vi "Parse All Elements.vi"(0 "Node in":refnum<k20>, 11 "error in":errorcluster) -> (4 "Node out":refnum<k20>, 6 "Section Data":T1, 8 "Child Items":cluster{"Item Type":T2, "Value":variant}[](array[cluster]), 10 "Properties out":refnum<class "Property.lvclass">[](array[class]), 15 "error out":errorcluster)   [LabVIEW 2024, in "Parser.lvlib" / "Section.lvclass"]
uses:
  Section.lvclass
  Item/Controls/Item Type.ctl
  Property/Property.lvclass
  <vilib>/xml/Close Reference(Node).vi
  <resource>/objmgr/DOMUserDefRef.rc
  <vilib>/xml/NI_XML.lvlib
  Channel/Channel.lvclass
  Item/Item.lvclass
  Parser.lvlib
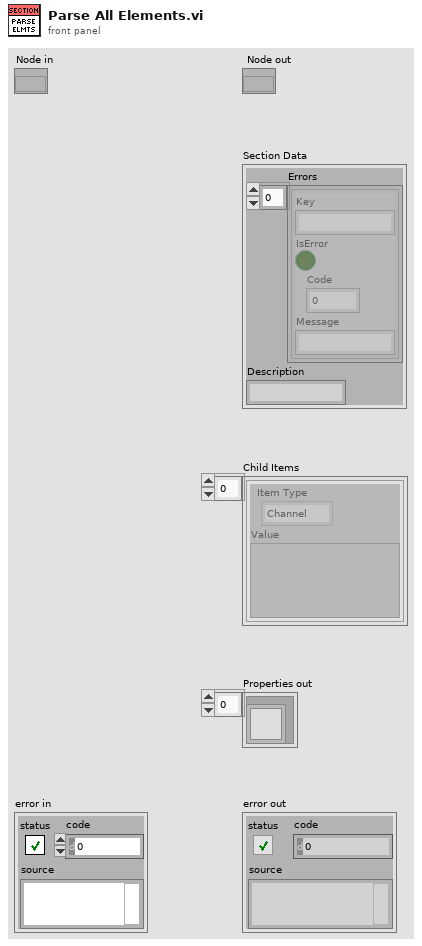
[diagram p1: front panel]
types:
  T1 = cluster{"Errors":cluster{"Key":string, "IsError":bool, "Code":u32, "Message":string}[], "Description":string}
  T2 = typedef "Parser.lvlib/Item.lvclass/Item Type.ctl" = enum16{"Channel", "Section"}
  T3 = cluster{"Key":string, "IsError":bool, "Code":u32, "Message":string}[]
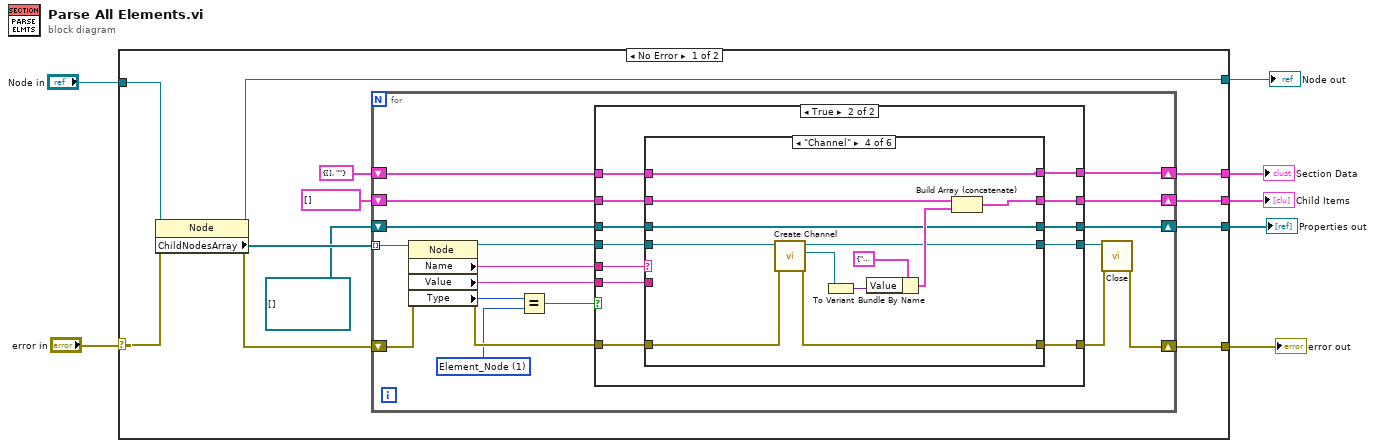
[diagram p0: block diagram]
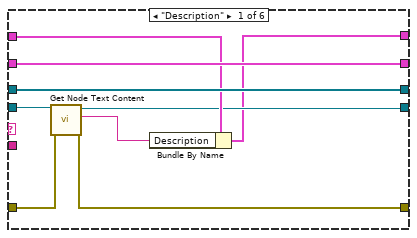
[diagram p3: hidden frame]
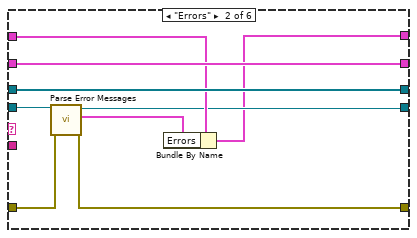
[diagram p4: hidden frame]
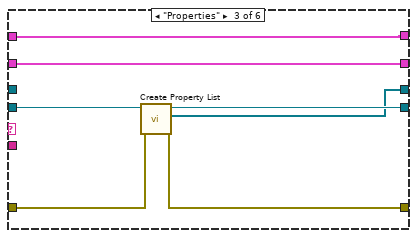
[diagram p5: hidden frame]
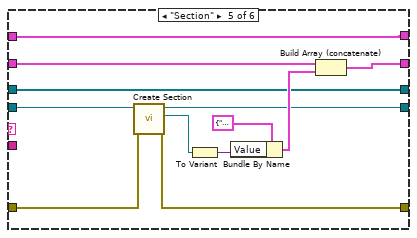
[diagram p6: hidden frame]
diagram:
  n1 = case shown="No Error" "error in" {
    selector: "error in" -> [w17 w109]
    tunnel: [w18 w109] -> w7
    tunnel: "Node in" -> [w16 _]
    tunnel: [w13 _] -> w4
    tunnel: [w11 _] -> w3
    tunnel: [w9 _] -> w2
    tunnel: [w8 _] -> w1
    frame No Error {
      n2 = property class="Node"(reference=w16, error in=w17) -> (reference out=w8:refnum<k20>, error out=w19:errorcluster, "ChildNodesArray"=w15:refnum<k20>[])
      n3 = for {
        tunnel: w15 -> [w33] mode=indexing
        shift-right: [w36] -> w18
        shift-left: w19 -> [w37]
        shift-right: [w24] -> w9
        shift-left: T1 {"Errors"=[], "Description"=""} ("Cluster of class private data") -> [w25]
        shift-right: [w22] -> w13
        shift-left: cluster{"Item Type":T2, "Value":variant}[] [] ("Child Items") -> [w23]
        shift-right: [w20] -> w11
        shift-left: refnum<class "Property.lvclass">[] [] ("reference out") -> [w21]
        w28 = 1 items=["Element_Node"=1, "Attribute_Node"=2, "Text_Node"=3, "CDATASection_Node"=4, "EntityReference_Node"=5, "Entity_Node"=6, "ProcessingInstruction_Node"=7, "Comment_Node"=8, "Document_Node"=9, "DocumentType_Node"=10, "DocumentFragment_Node"=11, "Notation_Node"=12] ("Node Type")
        n4 = property on="Property Node" class="Node"(reference=w33, error in=w37) -> (reference out=w31:refnum<k20>, error out=w35:errorcluster, "Name"=w32:string, "Value"=w30:string, "Type"=w26:i32)
        n5 = Equal?(x=w26, y=w28) -> (x = y?=w27:bool)
        n6 = case shown="True" w27 {
          tunnel: w32 -> [_ w52]
          tunnel: w31 -> [w41 w51]
          tunnel: w30 -> [_ w50]
          tunnel: [w41 w49] -> w29
          tunnel: w35 -> [w42 w54]
          tunnel: [w42 w53] -> w34
          tunnel: w25 -> [w40 w48]
          tunnel: [w40 w47] -> w24
          tunnel: w23 -> [w39 w46]
          tunnel: [w39 w45] -> w22
          tunnel: w21 -> [w38 w44]
          tunnel: [w38 w43] -> w20
          frame False {
          }
          frame True {
            n7 = case shown="\"Channel\"" w52 {
              tunnel: w51 -> [w58 w67 w77 w88 w100 w107]
              tunnel: w50 -> [_ _ _ _ _ _]
              tunnel: [w56 w66 w76 w80 w92 w107] -> w49
              tunnel: w54 -> [w63 w72 w79 w91 w103 w108]
              tunnel: [w62 w71 w78 w90 w102 w108] -> w53
              tunnel: w48 -> [w59 w68 w75 w89 w101 w106]
              tunnel: [w55 w64 w75 w89 w101 w106] -> w47
              tunnel: w46 -> [w61 w70 w73 w85 w97 w104]
              tunnel: [w61 w70 w73 w83 w95 w104] -> w45
              tunnel: w44 -> [w60 w69 _ w82 w94 w105]
              tunnel: [w60 w69 w74 w82 w94 w105] -> w43
              frame "Description" {
                n8 = call <vilib>:"Get Node Text Content.vi"("error in (no error)"=w63, "node in"=w58) -> ("error out"=w62:errorcluster, "node text"=w57:string, "node out"=w56:refnum<k20>)  [unwired: 7 in]
                n9 = Bundle By Name(cluster=w59, "Description"=w57) -> (w55:T1)
              }
              frame "Errors" {
                n10 = call "Parse Error Messages.vi"("error in"=w72, "Node in"=w67) -> ("error out"=w71:errorcluster, "Errors"=w65:T3, "Node out"=w66:refnum<k20>)  [unwired: 7 in]
                n11 = Bundle By Name(cluster=w68, "Errors"=w65) -> (w64:T1)
              }
              frame "Properties" {
                n12 = call "Create Property List.vi"("error in"=w79, "Property Nodes In"=w77) -> ("error out"=w78:errorcluster, "Properties out"=w74:refnum<class "Property.lvclass">[], "Property Nodes out"=w76:refnum<k20>)  [unwired: 7 in]
              }
              frame "Channel" {
                n13 = call "Create Channel.vi"("error in"=w91, "Node In"=w88) -> ("error out"=w90:errorcluster, "Channel out"=w81:refnum<class "Channel.lvclass">, "Node out"=w80:refnum<k20>)  [unwired: 7 in]
                n14 = To Variant(anything=w81) -> (Variant=w86:variant)
                n15 = Bundle By Name(cluster=cluster{"Item Type":T2, "Value":variant} {"Item Type"=enum."Channel", "Value"=variant} ("Child Items"), "Value"=w86) -> (w84:cluster{"Item Type":T2, "Value":variant})
                n16 = Build Array (concatenate)(w85, w84) -> (w83:cluster{"Item Type":T2, "Value":variant}[])
              }
              frame "Section" {
                n17 = call "Create Section.vi"("error in"=w103, "Node In"=w100) -> ("error out"=w102:errorcluster, "Section out"=w93:refnum<class "Section.lvclass">, "Node out"=w92:refnum<k20>)  [unwired: 7 in]
                n18 = To Variant(anything=w93) -> (Variant=w98:variant)
                n19 = Bundle By Name(cluster=cluster{"Item Type":T2, "Value":variant} {"Item Type"=enum."Section", "Value"=variant} ("Child Items"), "Value"=w98) -> (w96:cluster{"Item Type":T2, "Value":variant})
                n20 = Build Array (concatenate)(w97, w96) -> (w95:cluster{"Item Type":T2, "Value":variant}[])
              }
              frame "-1", Default {
              }
            }
          }
        }
        n21 = call-poly <vilib>:"Close.vi"("error in (no error)"=w34, "node"=w29) -> ("error out"=w36:errorcluster)  [unwired: 7 in]
      }
    }
    frame Error {
    }
  }
  "error out" <- w7
  "Child Items" <- w4
  "Properties out" <- w3
  "Section Data" <- w2
  "Node out" <- w1
